vi "Nextion_JacksInput_UART.vi"() -> (12 "b7":bool, 13 "b8":bool, 14 "b1":bool, 15 "b2":bool, 16 "b3":bool, 17 "b4":bool, 18 "b5":bool, 19 "b6":bool)   [LabVIEW 2019]
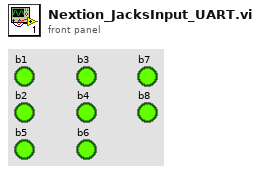
[diagram p1: front panel]
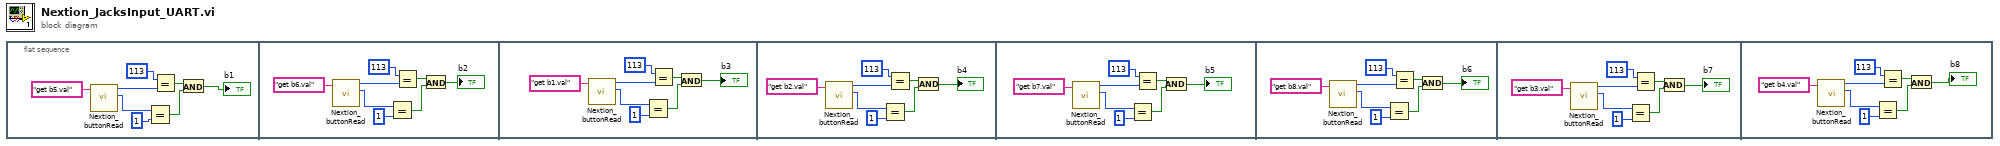
[diagram p0: block diagram]
diagram:
  n1 = flat-sequence {
    frame #0 {
      n2 = call "Nextion_buttonRead.vi"("string"="get b5.val") -> ("Bt_val"=w8:u8, "ref"=w7:u8)  [unwired: 8 in, 1 out]
      n3 = Equal?(x=w8, y=u8 1) -> (x = y?=w6:bool)
      n4 = Equal?(x=u8 113, y=w7) -> (x = y?=w5:bool)
      n5 = And(x=w5, y=w6) -> (x .and. y?=→"b1":bool)
    }
    frame #1 {
      n6 = call "Nextion_buttonRead.vi"("string"="get b6.val") -> ("Bt_val"=w12:u8, "ref"=w13:u8)  [unwired: 8 in, 1 out]
      n7 = Equal?(x=w12, y=u8 1) -> (x = y?=w14:bool)
      n8 = Equal?(x=u8 113, y=w13) -> (x = y?=w15:bool)
      n9 = And(x=w15, y=w14) -> (x .and. y?=→"b2":bool)
    }
    frame #2 {
      n10 = call "Nextion_buttonRead.vi"("string"="get b1.val") -> ("Bt_val"=w20:u8, "ref"=w21:u8)  [unwired: 8 in, 1 out]
      n11 = Equal?(x=w20, y=u8 1) -> (x = y?=w22:bool)
      n12 = Equal?(x=u8 113, y=w21) -> (x = y?=w23:bool)
      n13 = And(x=w23, y=w22) -> (x .and. y?=→"b3":bool)
    }
    frame #3 {
      n14 = call "Nextion_buttonRead.vi"("string"="get b2.val") -> ("Bt_val"=w28:u8, "ref"=w29:u8)  [unwired: 8 in, 1 out]
      n15 = Equal?(x=w28, y=u8 1) -> (x = y?=w30:bool)
      n16 = Equal?(x=u8 113, y=w29) -> (x = y?=w31:bool)
      n17 = And(x=w31, y=w30) -> (x .and. y?=→"b4":bool)
    }
    frame #4 {
      n18 = call "Nextion_buttonRead.vi"("string"="get b7.val") -> ("Bt_val"=w36:u8, "ref"=w37:u8)  [unwired: 8 in, 1 out]
      n19 = Equal?(x=w36, y=u8 1) -> (x = y?=w38:bool)
      n20 = Equal?(x=u8 113, y=w37) -> (x = y?=w39:bool)
      n21 = And(x=w39, y=w38) -> (x .and. y?=→"b5":bool)
    }
    frame #5 {
      n22 = call "Nextion_buttonRead.vi"("string"="get b8.val") -> ("Bt_val"=w44:u8, "ref"=w45:u8)  [unwired: 8 in, 1 out]
      n23 = Equal?(x=w44, y=u8 1) -> (x = y?=w46:bool)
      n24 = Equal?(x=u8 113, y=w45) -> (x = y?=w47:bool)
      n25 = And(x=w47, y=w46) -> (x .and. y?=→"b6":bool)
    }
    frame #6 {
      n26 = call "Nextion_buttonRead.vi"("string"="get b3.val") -> ("Bt_val"=w52:u8, "ref"=w53:u8)  [unwired: 8 in, 1 out]
      n27 = Equal?(x=w52, y=u8 1) -> (x = y?=w54:bool)
      n28 = Equal?(x=u8 113, y=w53) -> (x = y?=w55:bool)
      n29 = And(x=w55, y=w54) -> (x .and. y?=→"b7":bool)
    }
    frame #7 {
      n30 = call "Nextion_buttonRead.vi"("string"="get b4.val") -> ("Bt_val"=w60:u8, "ref"=w61:u8)  [unwired: 8 in, 1 out]
      n31 = Equal?(x=w60, y=u8 1) -> (x = y?=w62:bool)
      n32 = Equal?(x=u8 113, y=w61) -> (x = y?=w63:bool)
      n33 = And(x=w63, y=w62) -> (x .and. y?=→"b8":bool)
    }
  }
